vi "Process Monitor.vi"() -> ()   [LabVIEW 2014, in "SLL Process Monitor.lvlib"]
uses:
  SLL Process Monitor.lvlib
  <vilib>/Utility/error.llb/DialogType.ctl
  <vilib>/SLL/SLL Queued State Machine/Queue Driver/Create Queue.vi
  <vilib>/SLL/SLL Queued State Machine/Queue Driver/Enqueue an Item to Queue.vi
  <vilib>/SLL/SLL Queued State Machine/Queue Driver/Dequeue Queue.vi
  <vilib>/SLL/SLL Queued State Machine/Queue Driver/Enqueue N Items.vi
  <vilib>/SLL/SLL Queued State Machine/Queue Driver/Flush Queue.vi
  <vilib>/SLL/SLL Queued State Machine/Queue Driver/Release Queue.vi
  <vilib>/SLL/SLL Queued State Machine/SLL QSM.lvlib
panel:
  in  "Sampling Rate (s)":dbl=1.0
  in  "Application Image Name":string="LabVIEW"
  out "Waveform Chart":T1(graph)
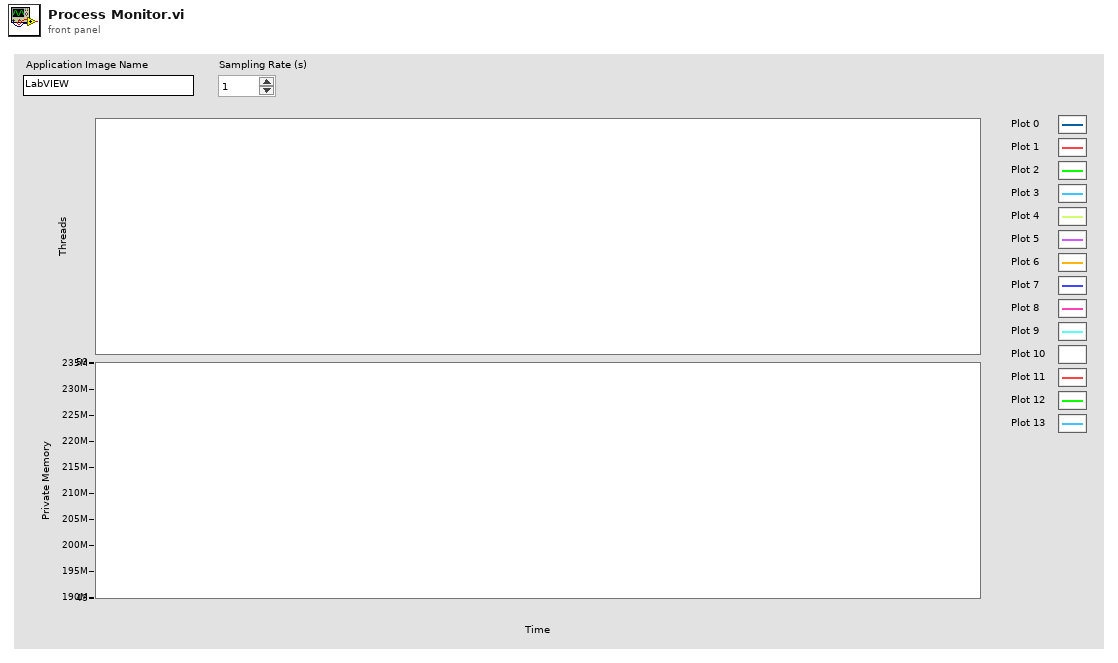
[diagram p1: front panel]
types:
  T1 = cluster{"Thread Count":i32, "PrivateMemorySize64":i64}
  T2 = cluster{"Flags":cluster{"Source Code?":bool}, "Application Name":string, "Ref":cluster{"ProcessMain":refnum<k24>, "UserProcess":refnum<k24>, "Threads":refnum<k24>}, "Sampling Rate (ms)":i32}
  T3 = cluster{"Thread Count":i32, "PrivateMemorySize64":i64}[]
  T4 = typedef "DialogType.ctl" = u16
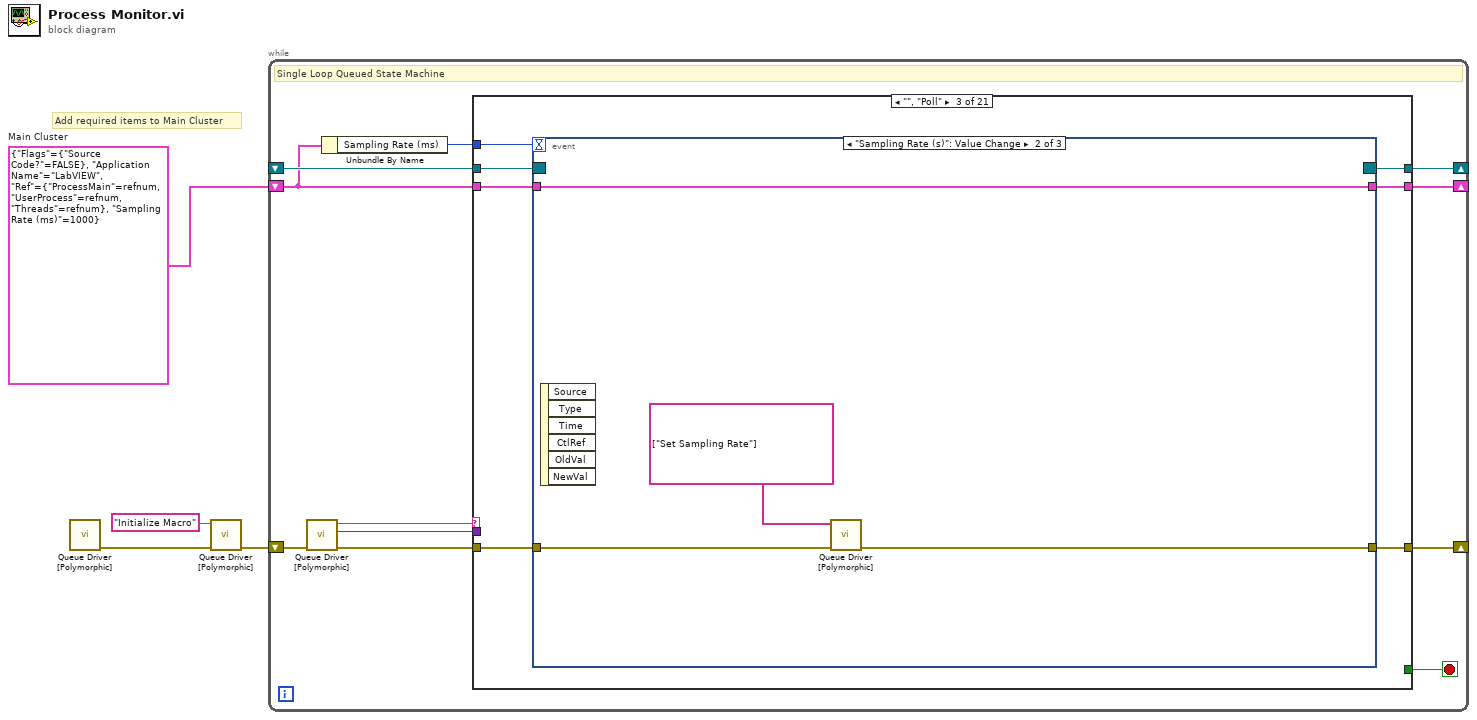
[diagram p0: block diagram]
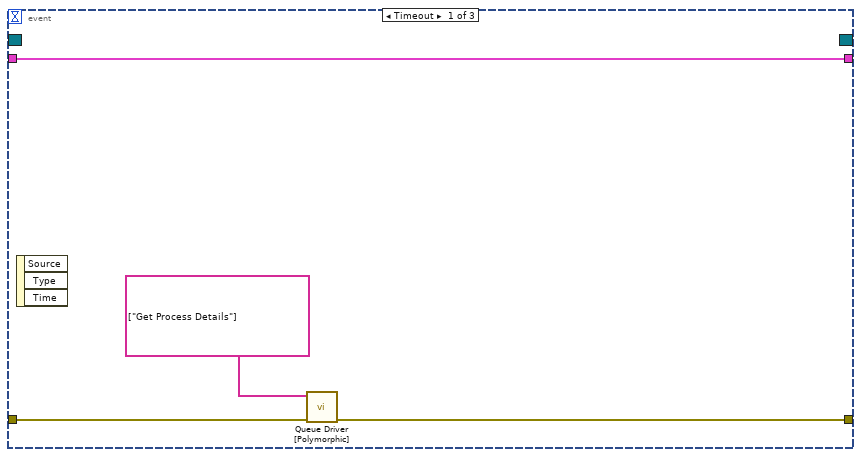
[diagram p4: hidden frame]
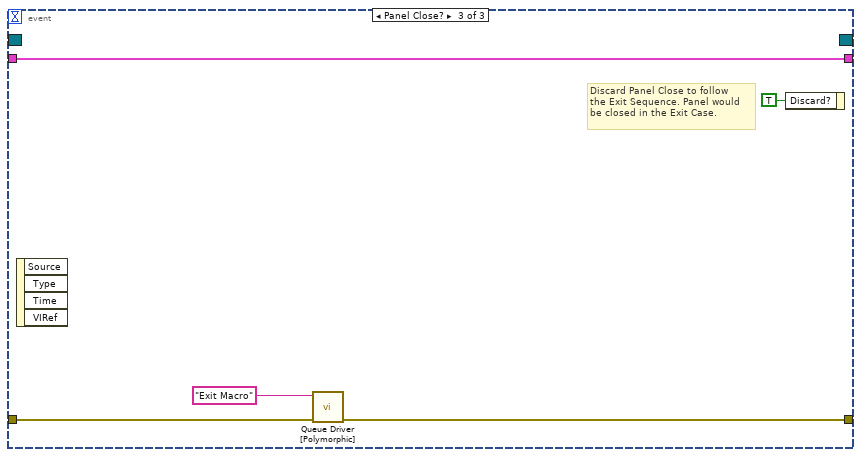
[diagram p5: hidden frame]
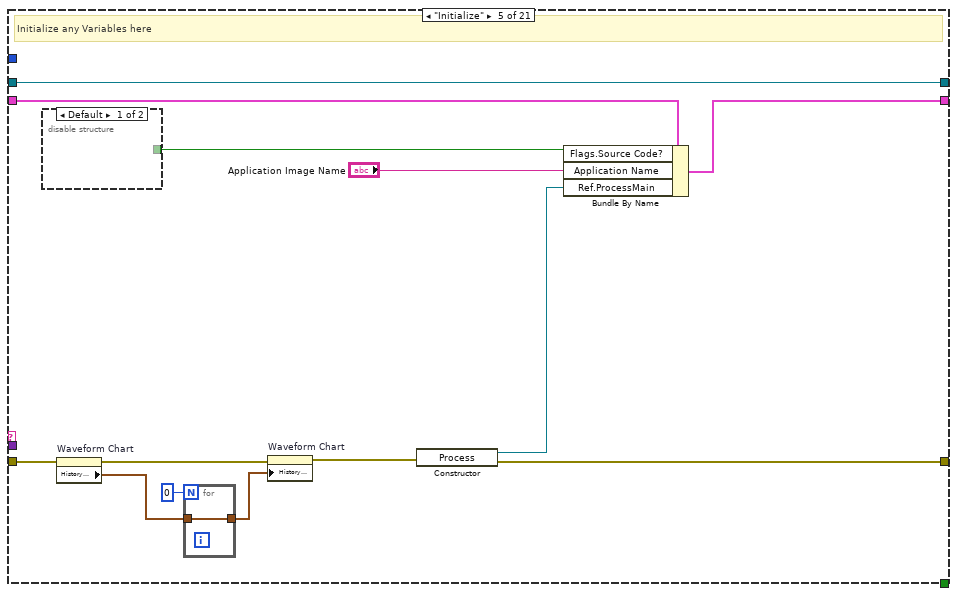
[diagram p7: hidden frame]
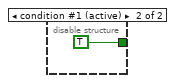
[diagram p8: hidden frame]
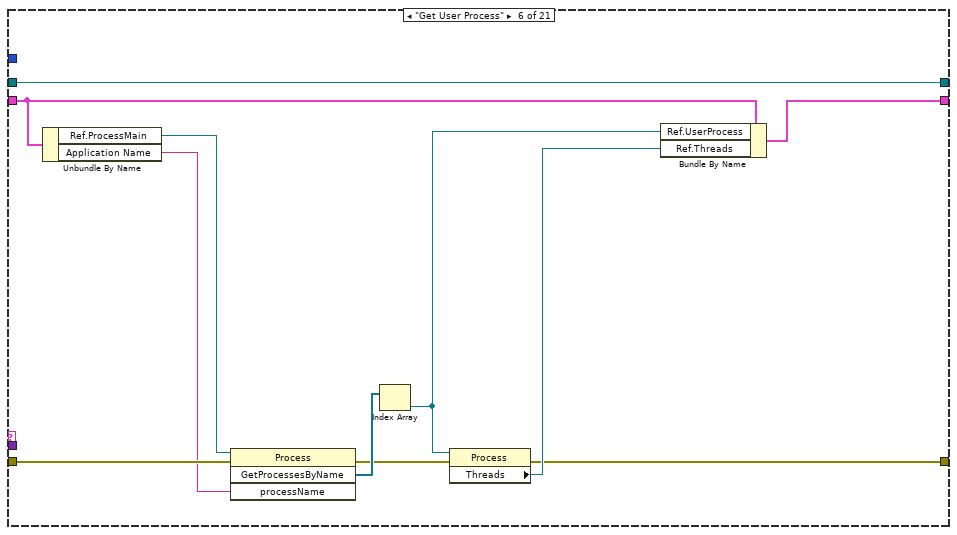
[diagram p9: hidden frame]
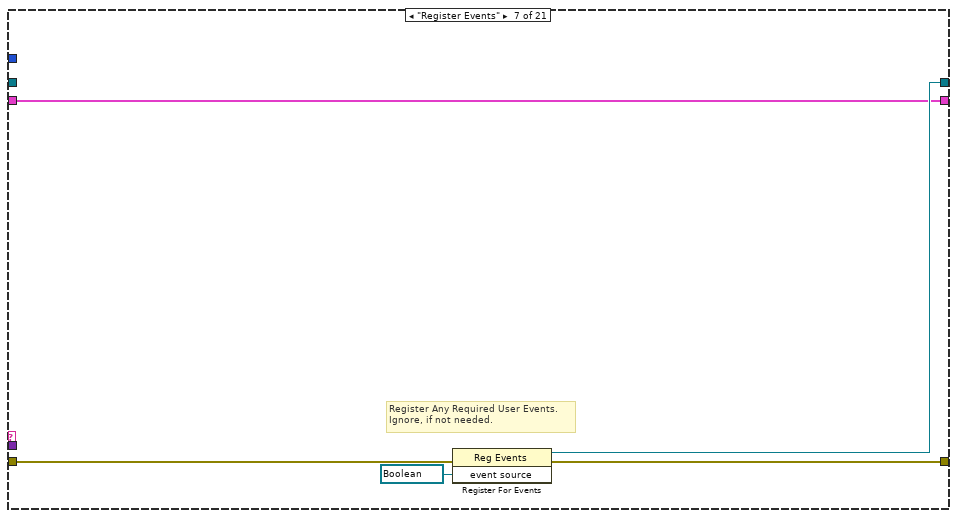
[diagram p10: hidden frame]
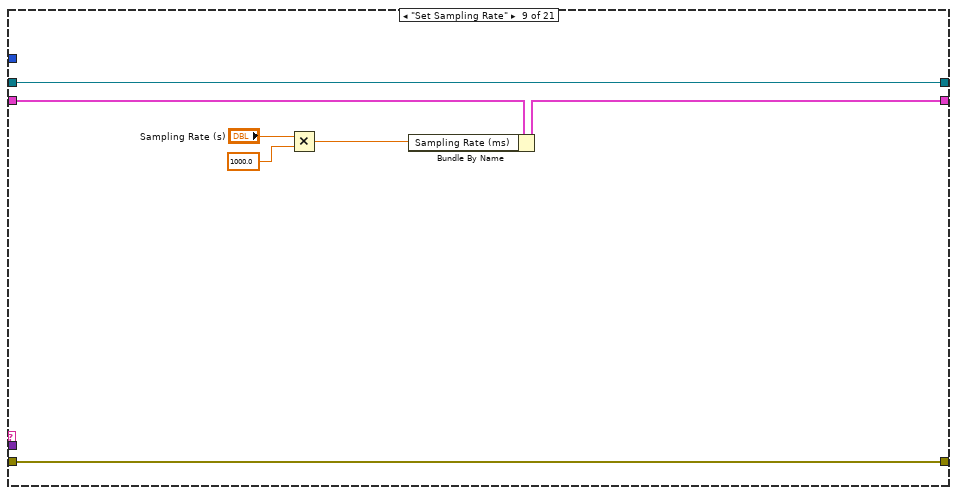
[diagram p12: hidden frame]
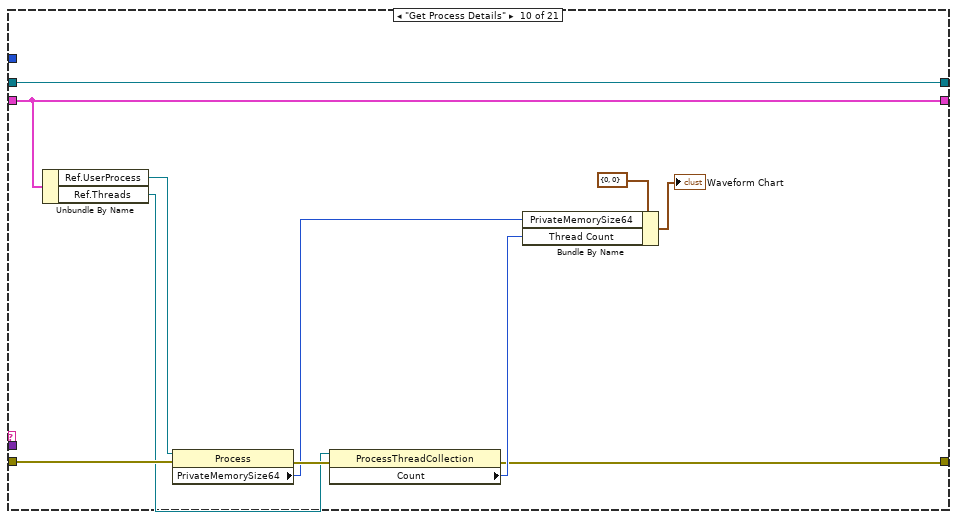
[diagram p13: hidden frame]
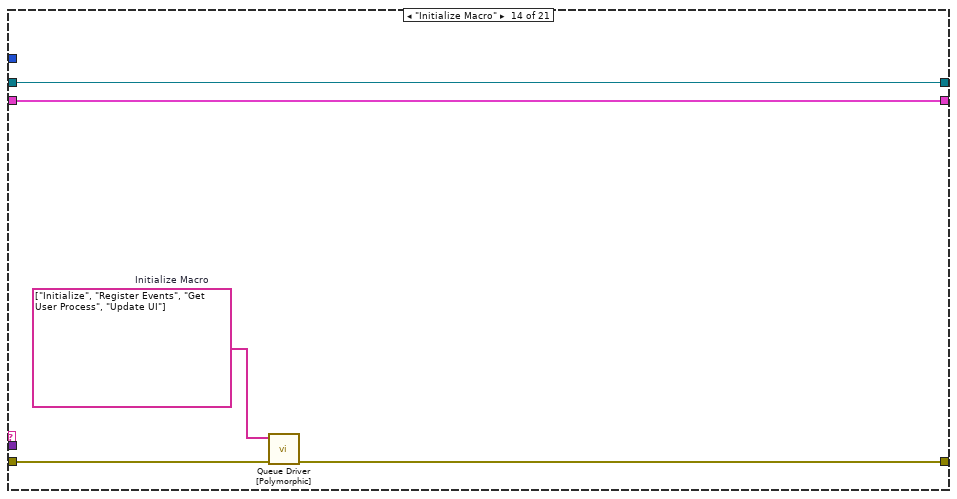
[diagram p17: hidden frame]
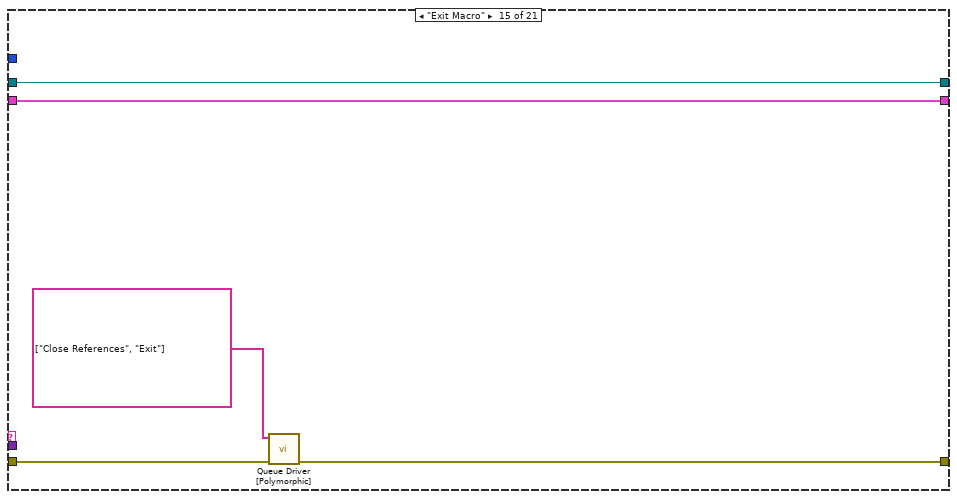
[diagram p18: hidden frame]
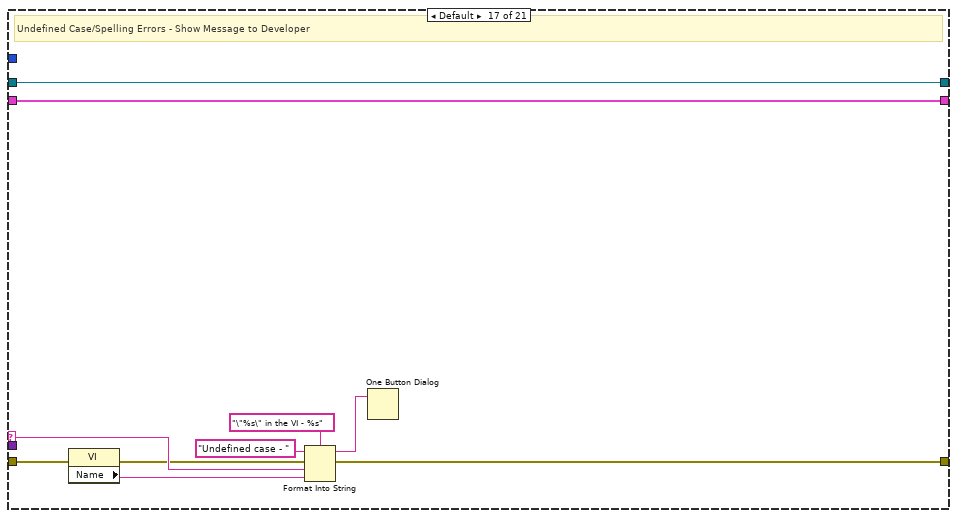
[diagram p20: hidden frame]
diagram:
  w3 = T2 {"Flags"={"Source Code?"=FALSE}, "Application Name"="LabVIEW", "Ref"={"ProcessMain"=refnum, "UserProcess"=refnum, "Threads"=refnum}, "Sampling Rate (ms)"=1000}  # Main Cluster
  # "Add required items to Main Cluster"
  n1 = call-poly <vilib>:"Queue Driver [Polymorphic].vi"() -> ("Error Out"=w1:errorcluster)  [unwired: 11 in]
  n2 = call-poly <vilib>:"Queue Driver [Polymorphic].vi"("Error In"=w1, "Item to Add"="Initialize Macro") -> ("Error Out"=w2:errorcluster)  [unwired: 9 in]
  n3 = while "SLL Queued State Machine" {
    shift-right: [w13] -> _
    shift-left: w2 -> [w15]
    shift-right: [w10] -> _
    shift-left: _ -> [w9]
    shift-right: [w8] -> _
    shift-left: w3 -> [w6]
    stop <- w12 stop-if-true
    # "Single Loop Queued State Machine"
    n4 = call-poly <vilib>:"Queue Driver [Polymorphic].vi"("Error In"=w15) -> ("Error Out"=w14:errorcluster, "Data"=w7:variant, "Dequeue"=w11:string)  [unwired: 8 in]
    n5 = Unbundle By Name(w6) -> ("Sampling Rate (ms)"=w5:i32)
    n6 = case "QSM Case Structure" shown="\"\", \"Poll\"" w11 {
      selector: w11 -> [_ _ _ _ _ _ _ _ _ _ _ _ _ _ _ _ w122 _ _ _ _]
      tunnel: w14 -> [w18 w21 w27 w44 w50 w67 w75 w78 w85 w94 w99 w102 w105 w108 w113 w118 w121 w134 w137 w139 w155]
      tunnel: [w18 w21 w28 w44 w52 w61 w74 w78 w85 w86 w99 w102 w105 w107 w112 w118 w125 w132 w137 w138 w151] -> w13
      tunnel: [_ _ _ _ _ _ _ _ _ _ _ _ _ _ _ _ _ _ _ _ TRUE] -> w12
      tunnel: [w17 w20 w26 w43 w57 w70 w73 w77 w84 w96 w98 w101 w104 w110 w115 w117 w128 w131 w136 w144 w154] -> w10
      tunnel: w9 -> [w17 w20 w25 w43 w57 w70 _ w77 w84 w96 w98 w101 w104 w110 w115 w117 w128 w131 w136 w144 w154]
      tunnel: [w16 w19 w23 w42 w54 w64 w72 w76 w80 w95 w97 w100 w103 w109 w114 w116 w127 w130 w135 w143 w153] -> w8
      tunnel: w6 -> [w16 w19 w24 w42 w55 w65 w72 w76 w83 w95 w97 w100 w103 w109 w114 w116 w127 w130 w135 w143 w153]
      tunnel: w7 -> [_ _ _ _ _ _ _ _ _ _ _ _ _ _ _ _ _ _ _ _ _]
      tunnel: w5 -> [_ _ w22 _ _ _ _ _ _ _ _ _ _ _ _ _ _ _ _ _ _]
      frame "/--------------- Read Me -----------------/" {
        # "General Purpose Queue Based State Machine for Any Use Case (main application, module, pop up message etc)\n\nAdvantages:\n1. No Need to Pass Queue References between Queue Driver VIs.\n2. This template can be safely used in multiple parallel running modules without any issues.\n3. This template can also be safely used even in cases where the VI is configured to be a Clone, where multiple \ninstances of the VI could be executing concurrently.\n\nHow to Use:\n1. Add necessary items to the Main Cluster.\n2. Use the Polymorphic Queue Driver for doing any queue operations. There is no need to pass the queue driver\nreference, as the Queue Driver automatically infers the reference based on the VI instance from which it is called.\n3. Add any required user events in the \"Register Events\" case. Ignore if not needed.\n4. Use \"Sequences\" section for defining any list of state calls, which could be used in multiple places. \nEg: Initialize Sequence, might be needed if we need to any reinitialization."
      }
      frame "/------------------ Poll -------------------/" {
      }
      frame "", "Poll" {
        n7 = event shown="[1] \"Sampling Rate (s)\": Value Change" {
          selector: w25 -> [_ _ _]
          dyn-events: [_ _ _] -> w26
          timeout: w22 -> [_ _ _]
          tunnel: [w30 w34 w40] -> w28
          tunnel: w27 -> [w31 w35 w41]
          tunnel: w24 -> [w32 w36 w39]
          tunnel: [w32 w36 w39] -> w23
          event Timeout {
            n8 = event-data() -> ()  [unwired: 1 in, 3 out]
            n9 = call-poly <vilib>:"Queue Driver [Polymorphic].vi"("Error In"=w31, "Enqueue N"=string[] ["Get Process Details"]) -> ("Error Out"=w30:errorcluster)  [unwired: 9 in]
          }
          event "Sampling Rate (s)": Value Change {
            n10 = event-data() -> ()  [unwired: 1 in, 6 out]
            n11 = call-poly <vilib>:"Queue Driver [Polymorphic].vi"("Error In"=w35, "Enqueue N"=string[] ["Set Sampling Rate"]) -> ("Error Out"=w34:errorcluster)  [unwired: 9 in]
          }
          event Panel Close? {
            # "Discard Panel Close to follow\nthe Exit Sequence. Panel would\nbe closed in the Exit Case."
            n12 = event-data() -> ()  [unwired: 1 in, 4 out]
            n13 = call-poly <vilib>:"Queue Driver [Polymorphic].vi"("Error In"=w41, "Item to Add"="Exit Macro" ("Enqueue")) -> ("Error Out"=w40:errorcluster)  [unwired: 9 in]
            n14 = event-data("Discard?"=TRUE) -> ()  [unwired: 1 in, 1 out]
          }
        }
      }
      frame "/--------------- Initialize -----------------/" {
      }
      frame "Initialize" {
        # "Initialize any Variables here"
        n15 = disable-structure shown="Default" {
          disable-tunnel: [_ TRUE] -> w56
          frame condition #0 {
          }
          frame condition #1 (active) {
          }
        }
        n16 = property on="Waveform Chart" class="WFChart (strict)"(error in=w50) -> (error out=w49:errorcluster, "History Data"=w46:T3)  [unwired: 1 in, 1 out]
        n17 = for {
          N: 0 -> [_]
          tunnel: w46 -> [w58]
          tunnel: [w58] -> w45
        }
        n18 = property on="Waveform Chart" class="WFChart (strict)"(error in=w49, "History Data"=w45) -> (error out=w48:errorcluster)  [unwired: 1 in, 1 out]
        n19 = constructor class="Process"(error in=w48) -> (reference out=w51:refnum<k24>, error out=w52:errorcluster)  [unwired: 2 in, 1 out]
        n20 = Bundle By Name(cluster=w55, "Flags.Source Code?"=w56, "Application Name"="Application Image Name", "Ref.ProcessMain"=w51) -> (w54:T2)
      }
      frame "Get User Process" {
        n21 = Unbundle By Name(w65) -> ("Ref.ProcessMain"=w68:refnum<k24>, "Application Name"=w66:string)
        n22 = invoke class="Process" method="GetProcessesByName"(reference=w68, error in=w67, "processName"=w66) -> (error out=w60:errorcluster, "GetProcessesByName"=w69:refnum<k24>[])  [unwired: 1 in, 2 out]
        n23 = Index Array(array=w69) -> (element=w63:refnum<k24>)  [unwired: 1 in]
        n24 = property class="Process"(reference=w63, error in=w60) -> (error out=w61:errorcluster, "Threads"=w62:refnum<k24>)  [unwired: 1 out]
        n25 = Bundle By Name(cluster=w65, "Ref.UserProcess"=w63, "Ref.Threads"=w62) -> (w64:T2)
      }
      frame "Register Events" {
        # "Register Any Required User Events. \nIgnore, if not needed."
        n26 = register-events(error in=w75, refnum<vi> refnum ("event source")) -> (reference out=w73:refnum<event-registration>, error out=w74:errorcluster)  [unwired: 1 in]
      }
      frame "/---------- Process Monitor ----------/" {
      }
      frame "Set Sampling Rate" {
        n27 = Multiply(x="Sampling Rate (s)", y=1000.0) -> (x*y=w79:dbl)
        n28 = Bundle By Name(cluster=w83, "Sampling Rate (ms)"=w79) -> (w80:T2)
      }
      frame "Get Process Details" {
        n29 = Unbundle By Name(w95) -> ("Ref.UserProcess"=w93:refnum<k24>, "Ref.Threads"=w90:refnum<k24>)
        n30 = property class="Process"(reference=w93, error in=w94) -> (error out=w92:errorcluster, "PrivateMemorySize64"=w89:i64)  [unwired: 1 out]
        n31 = property class="ProcessThreadCollection"(reference=w90, error in=w92) -> (error out=w86:errorcluster, "Count"=w88:i32)  [unwired: 1 out]
        n32 = Bundle By Name(cluster=T1 {"Thread Count"=0, "PrivateMemorySize64"=0}, "PrivateMemorySize64"=w89, "Thread Count"=w88) -> (→"Waveform Chart":T1)
      }
      frame "/-------------- User Interface --------------/" {
        # "Duplicate this case to create additional case splitters for readability"
      }
      frame "Update UI" {
        # "Update Front Panel Controls in this Case"
      }
      frame "/----------------- Macros -----------------/" {
      }
      frame "Initialize Macro" {
        w106 = string[] ["Initialize", "Register Events", "Get User Process", "Update UI"]  # Initialize Macro
        n33 = call-poly <vilib>:"Queue Driver [Polymorphic].vi"("Error In"=w108, "Enqueue N"=w106) -> ("Error Out"=w107:errorcluster)  [unwired: 9 in]
      }
      frame "Exit Macro" {
        n34 = call-poly <vilib>:"Queue Driver [Polymorphic].vi"("Error In"=w113, "Enqueue N"=string[] ["Close References", "Exit"]) -> ("Error Out"=w112:errorcluster)  [unwired: 9 in]
      }
      frame "/-------------- Error Handler--------------/" {
      }
      frame Default {
        # "Undefined Case/Spelling Errors - Show Message to Developer"
        n35 = property class="VI"(error in=w121) -> (error out=w120:errorcluster, "Name"=w119:string)  [unwired: 1 in, 1 out]
        n36 = Format Into String(format string="\"%s\" in the VI - %s" ("message"), initial string="Undefined case - ", error in=w120, w122, w119) -> (resulting string=w123:string, error out=w125:errorcluster)
        n37 = One Button Dialog(message=w123) -> ()  [unwired: 1 in, 1 out]
      }
      frame "Error" {
        w129 = T4 2 items=["no dialog", "OK message", "continue or stop message", "OK message + warnings", "continue/stop + warnings"] ("type of dialog (OK msg:1)")
        # "Handle the Error"
        n38 = call <vilib>:"Simple Error Handler.vi"("type of dialog (OK msg:1)"=w129, "error in (no error)"=w134) -> ("error out"=w133:errorcluster)  [unwired: 3 in, 4 out]
        n39 = call <vilib>:"Clear Errors.vi"("error in (no error)"=w133) -> ("error out"=w132:errorcluster)  [unwired: 5 in, 1 out]
      }
      frame "/------------------- Exit --------------------/" {
      }
      frame "Close References" {
        n40 = Unbundle By Name(w143) -> ("Ref.ProcessMain"=w140:refnum<k24>, "Ref.UserProcess"=w141:refnum<k24>)
        n41 = Close Reference(reference=w141, error in (no error)=w139) -> (error out=w142:errorcluster)
        n42 = Close Reference(reference=w140, error in (no error)=w142) -> (error out=w138:errorcluster)
      }
      frame "Exit" {
        n43 = call-poly <vilib>:"Queue Driver [Polymorphic].vi"("Error In"=w155) -> ("Error Out"=w156:errorcluster)  [unwired: 9 in, 1 out]
        n44 = Unbundle By Name(w153) -> ("Flags.Source Code?"=w146:bool)
        n45 = call-poly <vilib>:"Queue Driver [Polymorphic].vi"("Error In"=w156) -> ("Error Out"=w152:errorcluster)  [unwired: 10 in]
        n46 = Call Chain() -> (call chain=w150:string[])
        n47 = Array Size(array=w150) -> (size(s)=w149:i32)
        n48 = Equal?(x=w149, y=1) -> (x = y?=w147:bool)
        n49 = And(x=w146, y=w147) -> (x .and. y?=w145:bool)
        n50 = case "Skip Panel Close when in Source\nCode and is the top most caller" shown="True" w145 {
          tunnel: w152 -> [w159 w161]
          tunnel: [w160 w161] -> w151
          frame False {
            # "Close Panel"
            n51 = invoke class="VI" method="FP.Close"() -> (error out=w158:errorcluster)  [unwired: 3 in, 2 out]
            n52 = Merge Errors(w159, w158) -> (w160:errorcluster)
          }
          frame True {
            # "Do Not Close Panel"
          }
        }
      }
    }
  }
